vi "IsmaCTRL.vi"(1 "FR_manual":dbl, 8 "Manual":bool, 12 "Reset":bool, 14 "Pause":bool, 16 "Setpoint_W   /   Setpoint_T":dbl[][](array[numeric]), 18 "Enable":bool, 19 "Scale":dbl[](array[numeric])) -> (3 "Boolean 9":bool, 4 "Boolean":bool, 5 "Boolean 2":bool, 7 "Boolean 3":bool, 9 "Boolean 4":bool, 13 "Boolean 5":bool, 15 "Boolean 6":bool, 17 "Boolean 7":bool, 20 "FR":dbl, 21 "RPM":dbl, 22 "Weight":dbl, 23 "elapsed":dbl, 24 "time_to_target":dbl, 25 "pumpCTRL":dbl, 27 "Boolean 8":bool)   [LabVIEW 2017]
uses:
  BERTTA.dll
panel:
  out "paramsIn":dbl[](array[numeric])
  out "paramsOut":dbl[](array[numeric])
  # "STOP"
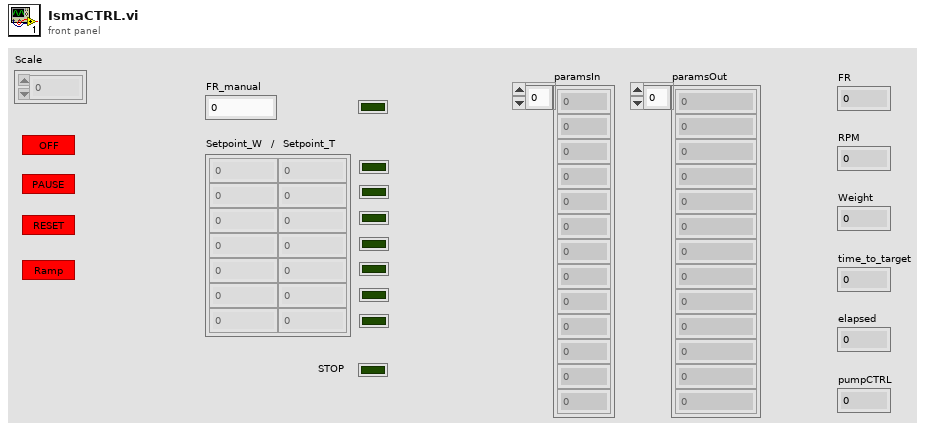
[diagram p1: front panel]
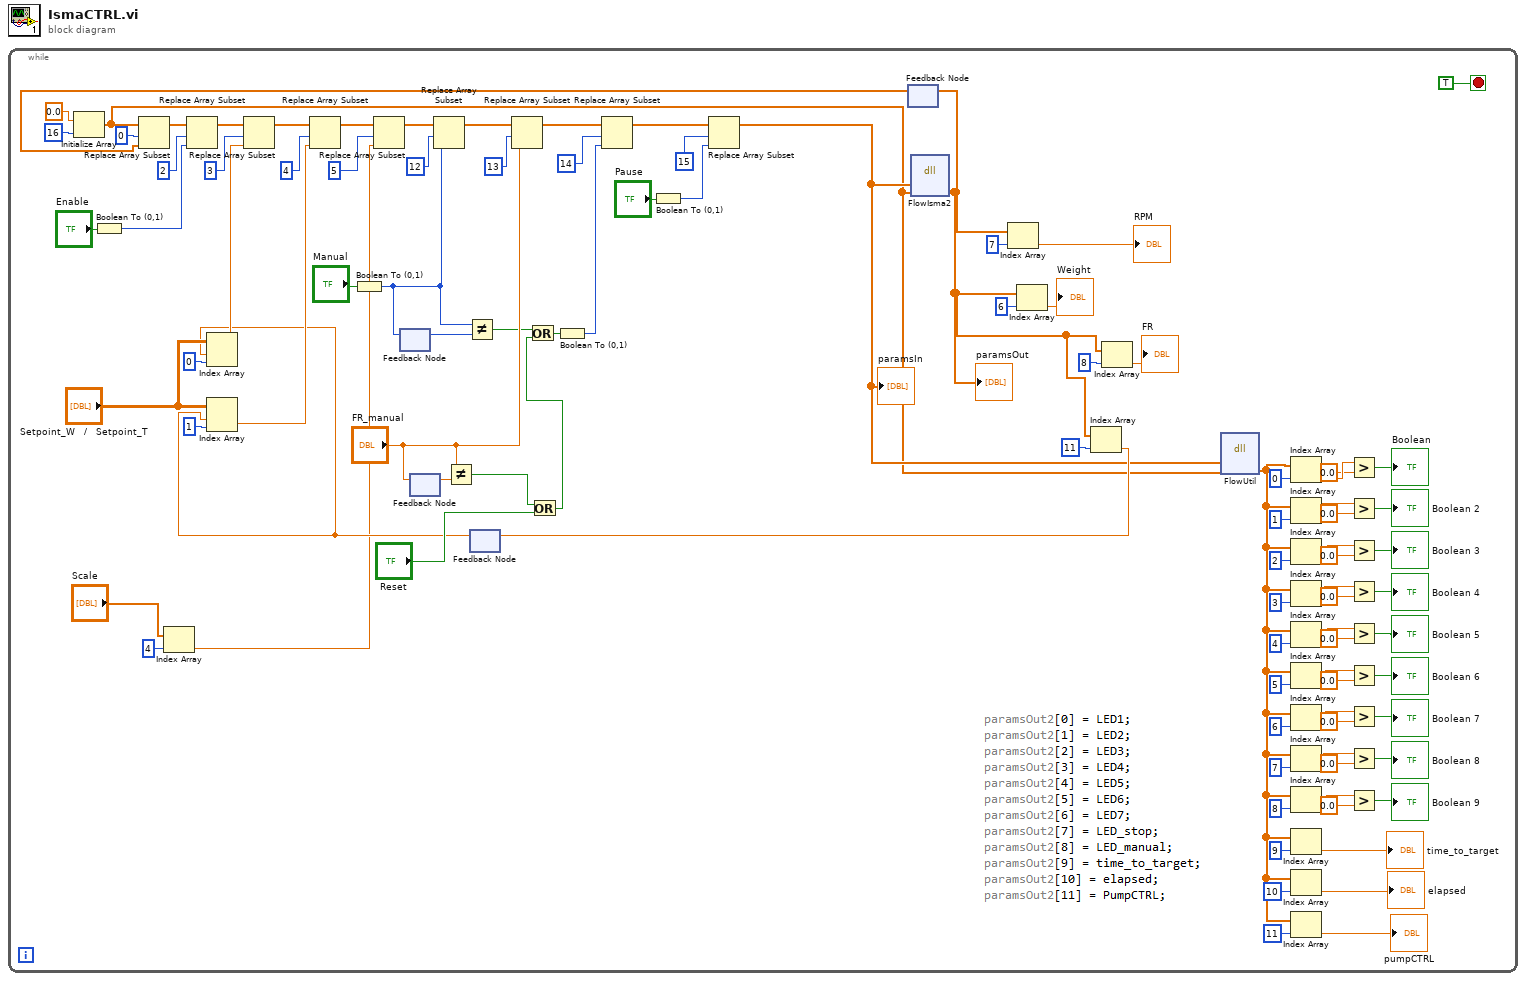
[diagram p0: block diagram]
diagram:
  n1 = while {
    stop <- TRUE stop-if-true
    n2 = Initialize Array(0.0 ("element"), 16 ("dimension size")) -> (w5:dbl[])
    n3 = Boolean To (0,1)(Boolean="Enable") -> (0, 1=w77:i16)
    n4 = Index Array(array="Scale", index=4) -> (element=w2:dbl)
    n5 = Boolean To (0,1)(Boolean="Manual") -> (0, 1=w68:i16)
    n6 = feedback #1() -> (w69:i16)  [unwired: 1 in]
    n7 = feedback-in #1(w68) -> ()
    n8 = feedback #2() -> (w72:dbl)  [unwired: 1 in]
    n9 = feedback-in #2("FR_manual") -> ()
    n10 = Not Equal?(x="FR_manual", y=w72) -> (x != y?=w71:bool)
    n11 = Not Equal?(x=w68, y=w69) -> (x != y?=w65:bool)
    n12 = feedback #3() -> (w50:dbl)  [unwired: 1 in]
    n13 = Index Array(array="Setpoint_W   /   Setpoint_T", index (row)=w50, index (col)=0 ("disabled index (col)")) -> (element=w57:dbl)
    n14 = Index Array(array="Setpoint_W   /   Setpoint_T", index (row)=w50, index (col)=1 ("disabled index (col)")) -> (element=w54:dbl)
    n15 = Or(x=w71, y="Reset") -> (x .or. y?=w64:bool)
    n16 = Or(x=w65, y=w64) -> (x .or. y?=w67:bool)
    n17 = Boolean To (0,1)(Boolean=w67) -> (0, 1=w66:i16)
    n18 = Boolean To (0,1)(Boolean="Pause") -> (0, 1=w59:i16)
    n19 = feedback #4() -> (w85:dbl[])  [unwired: 1 in]
    n20 = Replace Array Subset(array=w5, new element=w85, index=0) -> (w84:dbl[])
    n21 = Replace Array Subset(array=w84, new element=w77, index=2) -> (w94:dbl[])
    n22 = Replace Array Subset(array=w94, new element=w57, index=3) -> (w92:dbl[])
    n23 = Replace Array Subset(array=w92, new element=w54, index=4) -> (w90:dbl[])
    n24 = Replace Array Subset(array=w90, new element=w2, index=5) -> (w82:dbl[])
    n25 = Replace Array Subset(array=w82, new element=w68, index=12) -> (w79:dbl[])
    n26 = Replace Array Subset(array=w79, new element="FR_manual", index=13) -> (w74:dbl[])
    n27 = Replace Array Subset(array=w74, new element=w66, index=14) -> (w61:dbl[])
    n28 = Replace Array Subset(array=w61, new element=w59, index=15) -> (w49:dbl[])
    "paramsIn" <- w49
    n29 = dll-call lib="C:/Users/shresplab/OneDrive - Kemira Oyj/Documents/GitHub/Bertta/BERTTA/x64/Debug/BERTTA.dll" fn="FlowIsma2"("paramsIn"=w49, "paramsOut"=w5) -> ("paramsOut"=w52:dbl[])  [unwired: 5 in, 2 out]
    "paramsOut" <- w52
    n30 = feedback-in #4(w52) -> ()
    n31 = Index Array(array=w52, index=7) -> (element=→"RPM":dbl)
    n32 = Index Array(array=w52, index=6) -> (element=→"Weight":dbl)
    n33 = Index Array(array=w52, index=11) -> (element=w51:dbl)
    n34 = feedback-in #3(w51) -> ()
    n35 = Index Array(array=w52, index=8) -> (element=→"FR":dbl)
    n36 = dll-call lib="C:/Users/shresplab/OneDrive - Kemira Oyj/Documents/GitHub/Bertta/BERTTA/x64/Debug/BERTTA.dll" fn="FlowUtil"("paramsIn"=w49, "paramsOut2"=w5) -> ("paramsOut2"=w36:dbl[])  [unwired: 5 in, 2 out]
    n37 = Index Array(array=w36, index=0) -> (element=w35:dbl)
    n38 = Index Array(array=w36, index=1) -> (element=w34:dbl)
    n39 = Index Array(array=w36, index=2) -> (element=w33:dbl)
    n40 = Index Array(array=w36, index=3) -> (element=w32:dbl)
    n41 = Index Array(array=w36, index=4) -> (element=w31:dbl)
    n42 = Index Array(array=w36, index=5) -> (element=w30:dbl)
    n43 = Index Array(array=w36, index=6) -> (element=w29:dbl)
    n44 = Index Array(array=w36, index=7) -> (element=w28:dbl)
    n45 = Index Array(array=w36, index=8) -> (element=w27:dbl)
    n46 = Index Array(array=w36, index=9) -> (element=→"time_to_target":dbl)
    n47 = Index Array(array=w36, index=10) -> (element=→"elapsed":dbl)
    n48 = Index Array(array=w36, index=11) -> (element=→"pumpCTRL":dbl)
    n49 = Greater?(x=w35, y=0.0) -> (0:→"Boolean":bool)
    n50 = Greater?(x=w34, y=0.0) -> (0:→"Boolean 2":bool)
    n51 = Greater?(x=w33, y=0.0) -> (0:→"Boolean 3":bool)
    n52 = Greater?(x=w32, y=0.0) -> (0:→"Boolean 4":bool)
    n53 = Greater?(x=w31, y=0.0) -> (0:→"Boolean 5":bool)
    n54 = Greater?(x=w30, y=0.0) -> (0:→"Boolean 6":bool)
    n55 = Greater?(x=w29, y=0.0) -> (0:→"Boolean 7":bool)
    n56 = Greater?(x=w28, y=0.0) -> (0:→"Boolean 8":bool)
    n57 = Greater?(x=w27, y=0.0) -> (0:→"Boolean 9":bool)
  }
